vi "main_NI.vi"() -> ()   [LabVIEW 2017]
doc: "Эта версия для работы с системой сбора данных Agilent 34980A"
uses:
  <instrlib>/niDMM/nidmm.llb/niDMM Powerline Frequency.ctl
  <instrlib>/niDMM/nidmm.llb/niDMM Resolution in Digits.ctl
  <instrlib>/niDMM/nidmm.llb/niDMM Function.ctl
  <instrlib>/niDMM/nidmm.llb/niDMM Auto Zero.ctl
  <instrlib>/niDMM/nidmm.llb/niDMM ADC Calibration.ctl
  <vilib>/SwitchExecutive/nise.llb/niSE SessionRefnum.ctl
  <instrlib>/niDMM/nidmm.llb/niDMM Configure Measurement Digits.vi
  <vilib>/Utility/file.llb/Write Delimited Spreadsheet (string).vi
  VI/????????? ? ????????? ???????????? 34980A.vi
panel:
  in  "AllPlot":bool=TRUE caption="Все граф."
  out "Volt_3":dbl caption="V_3"
  in  "amountChip":i32=1 caption="Кол-во м/х" min=1 max=16 step=1
  out "isDMM":bool
  in  "DMM":refnum<k15>="-----"
  in  "wait befor meas, ms":u32=100 caption="Задержка ПЕРЕД\nизмерением, мс"
  out "ArrayTime 2":dbl[](array[numeric])
  out "Volt_2":dbl caption="V_2"
  out "Volt_1":dbl caption="V_1"
  in  "Emulate":bool
  out "ArrayOut":string[][](array[string])
  out "timer, s":dbl caption="Таймер, с"
  out "Waveform Graph":dbl[][](graph)
  in  "WaitAfterMeas, sec":u32 caption="Задержка ПОСЛЕ\nизм. всех приборов, с"
  in  "Record Data":bool
  out "error out":errorcluster
  in  "Save Button":bool
  # "В"
  # "В"
  # "В"
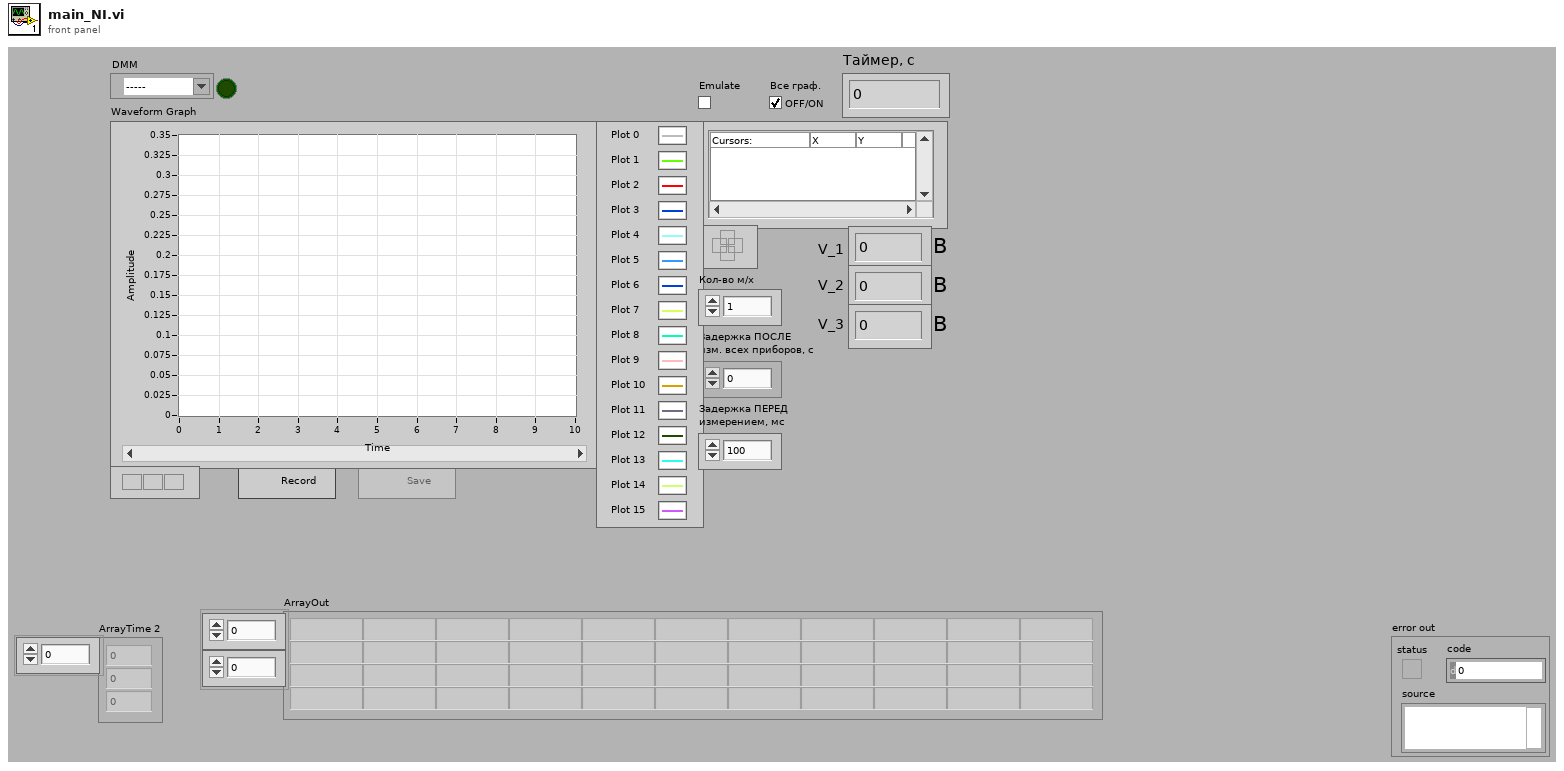
[diagram p1: front panel]
types:
  T1 = cluster{"Microchip_1":dbl[], "Microchip_2":dbl[], "Microchip_3":dbl[], "Microchip_4":dbl[], "Microchip_5":dbl[], "Microchip_6":dbl[], "Microchip_7":dbl[], "Microchip_8":dbl[], "Microchip_9":dbl[], "Microchip_10":dbl[], "Microchip_11":dbl[], "Microchip_12":dbl[], "Microchip_13":dbl[], "Microchip_14":dbl[], "Microchip_15":dbl[], "Microchip_16":dbl[]}
  T2 = enum8{"Enabled", "Disabled", "Disabled and Grayed Out"}
  T3 = typedef "niDMM Function.ctl" = enum16{"DC Volts", "AC Volts", "DC Current", "AC Current", "2-wire Resistance", "4-wire Resistance", "Diode", "Frequency", "Period", "AC Volts DC Coupled", "Capacitance", "Inductance", "Temperature"}
  T4 = typedef "niDMM Powerline Frequency.ctl" = enum16{"60 Hz", "50 Hz"}
  T5 = typedef "niDMM ADC Calibration.ctl" = i32
  T6 = typedef "niDMM Auto Zero.ctl" = i32
  T7 = typedef "niDMM Resolution in Digits.ctl" = dbl
  T8 = typedef "niSE SessionRefnum.ctl" = refnum<k1>
  T9 = cluster{"Microchip_1":string[], "Microchip_2":string[], "Microchip_3":string[], "Microchip_4":string[], "Microchip_5":string[], "Microchip_6":string[], "Microchip_7":string[], "Microchip_8":string[], "Microchip_9":string[], "Microchip_10":string[], "Microchip_11":string[], "Microchip_12":string[], "Microchip_13":string[], "Microchip_14":string[], "Microchip_15":string[], "Microchip_16":string[]}
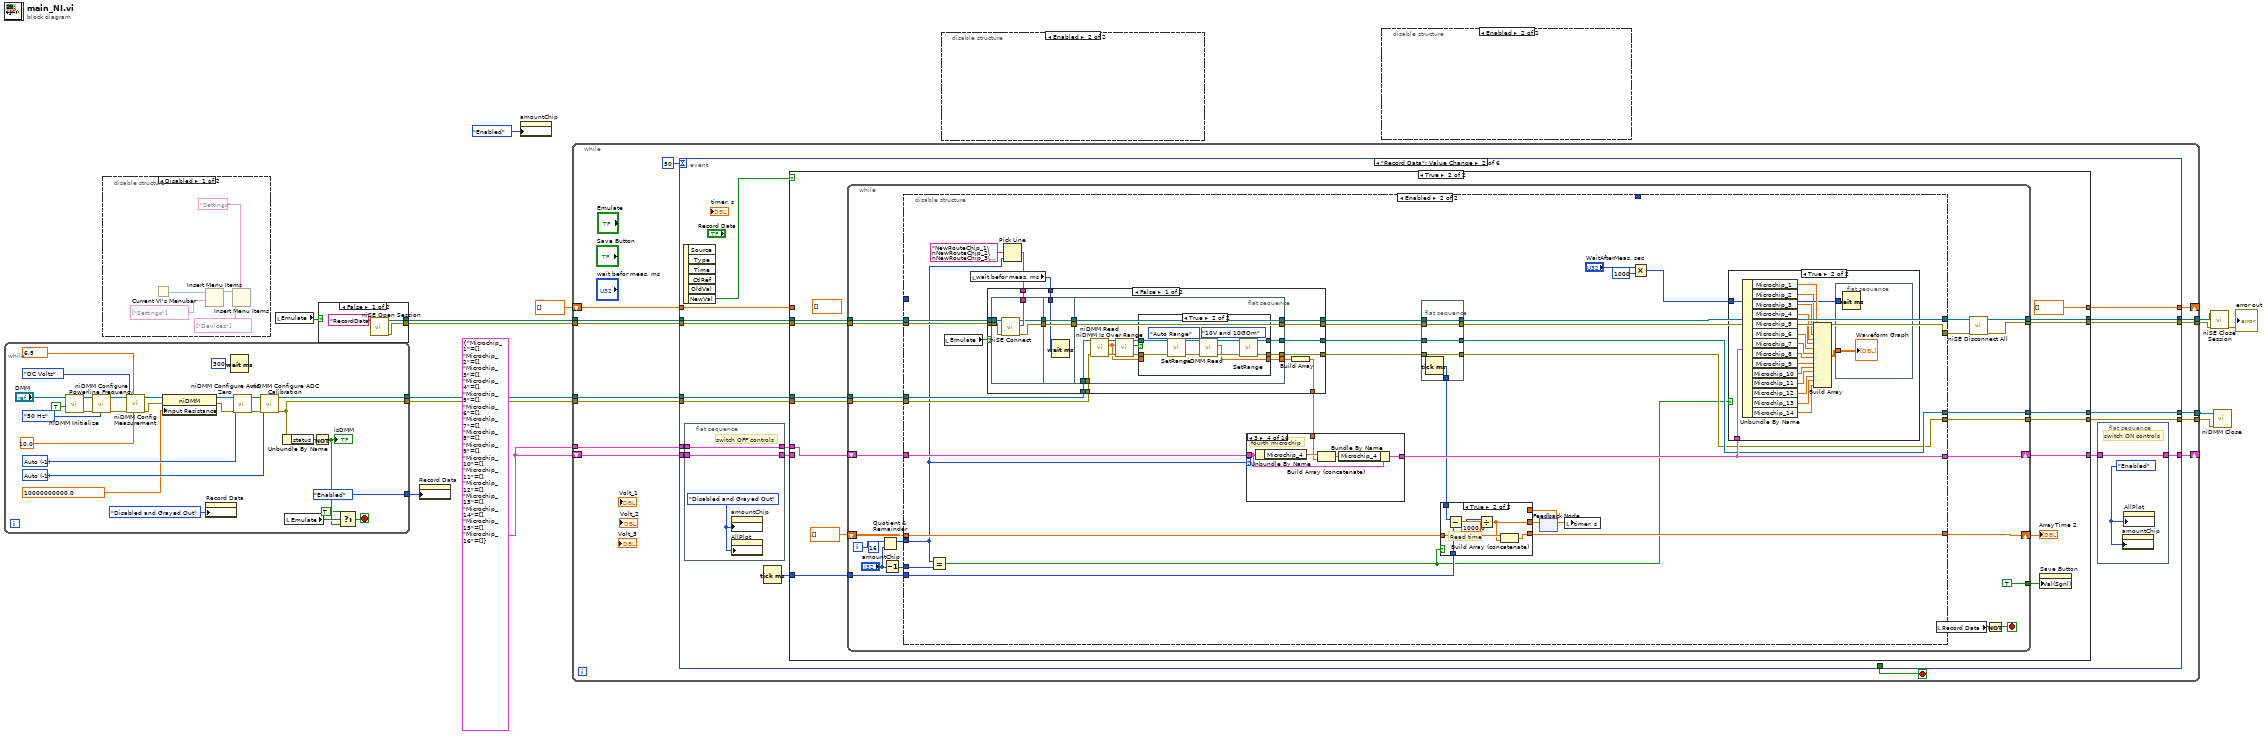
[diagram p0: block diagram]
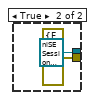
[diagram p2: hidden frame]
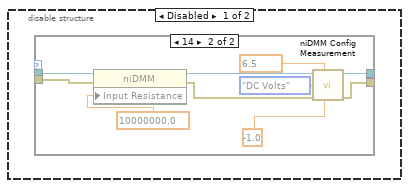
[diagram p3: hidden frame]
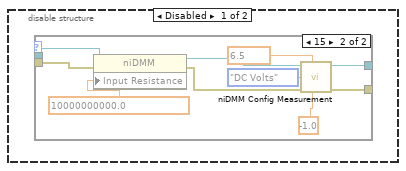
[diagram p5: hidden frame]
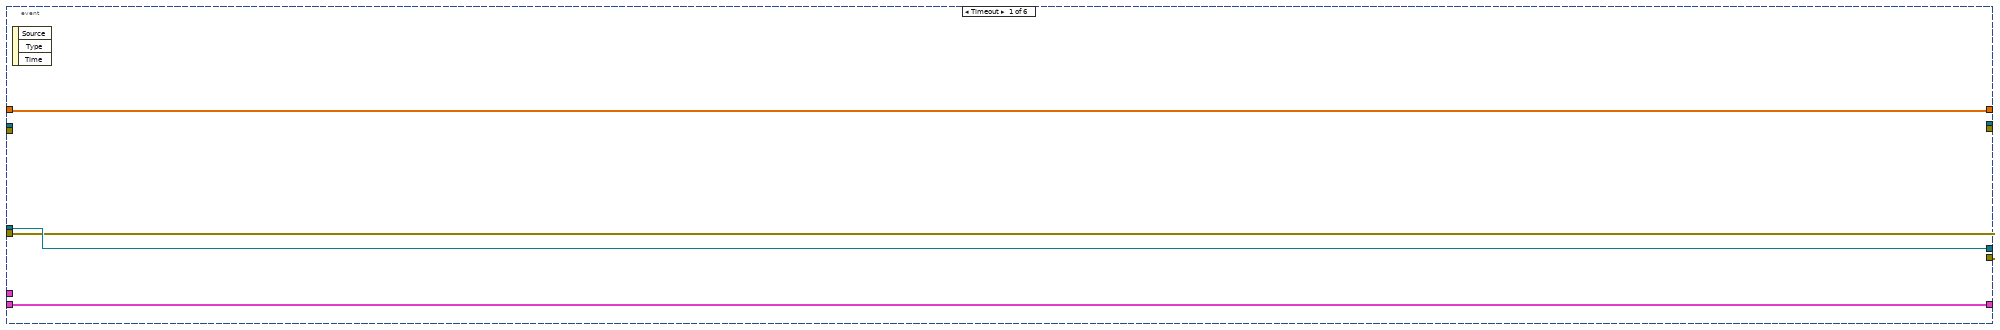
[diagram p8: hidden frame]
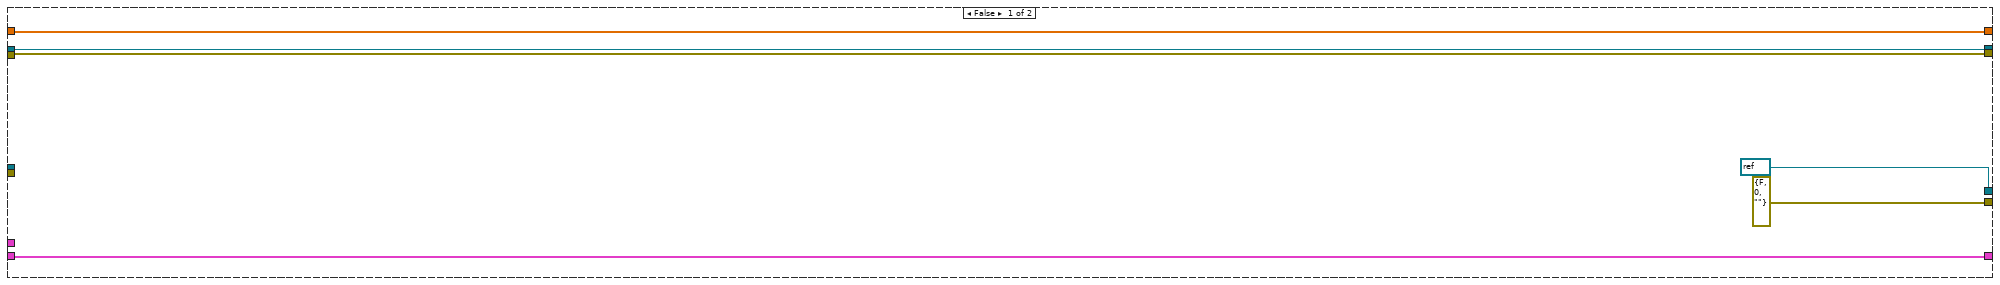
[diagram p9: hidden frame]
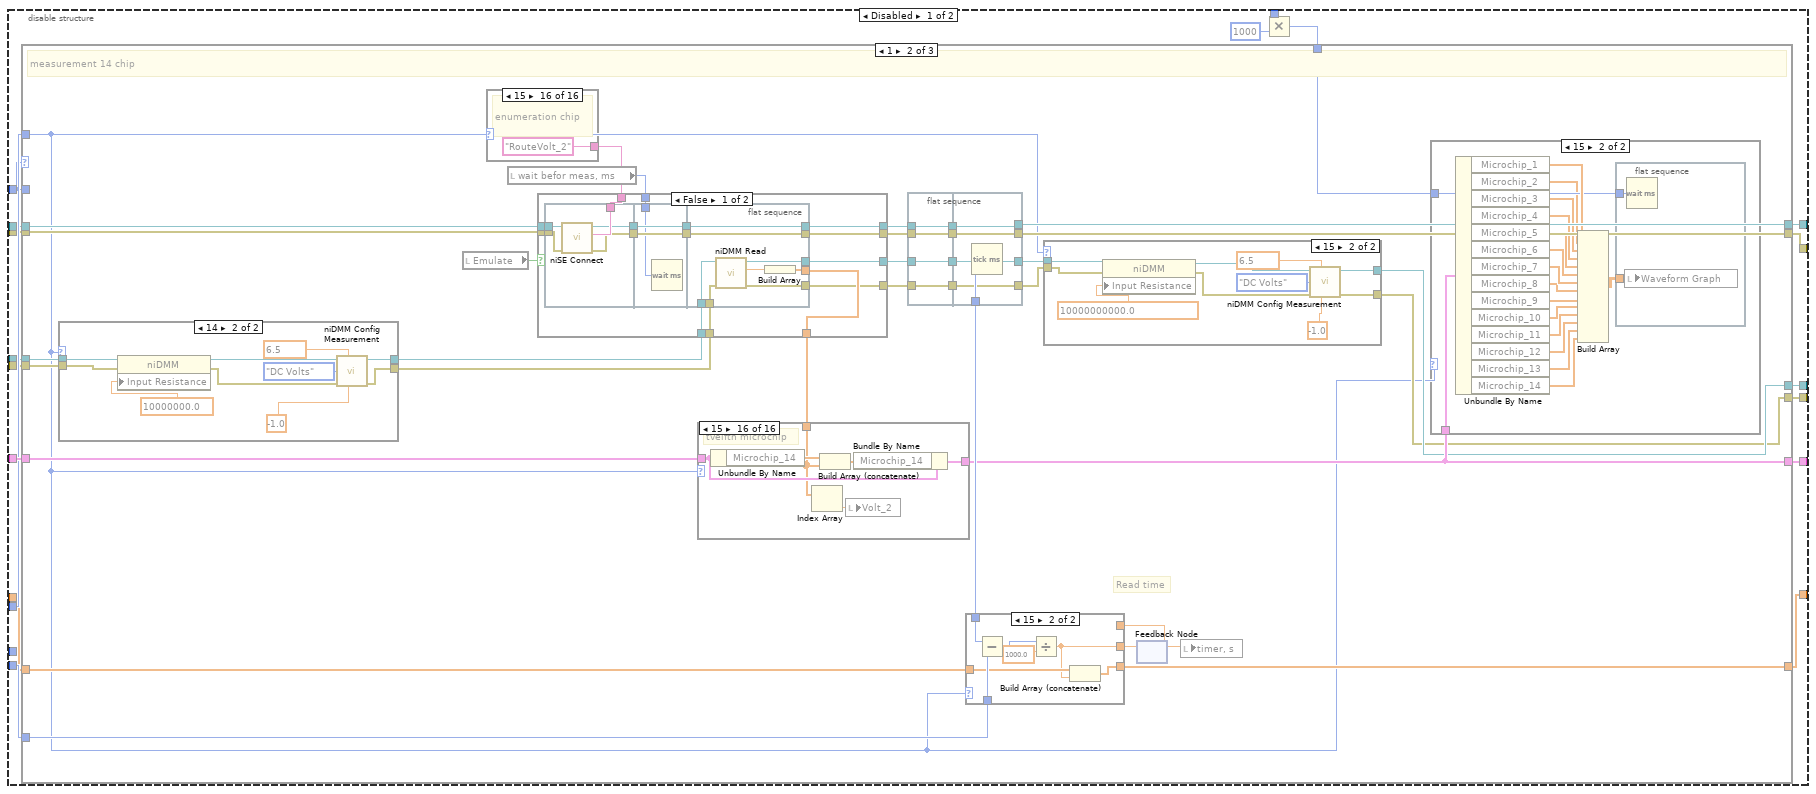
[diagram p10: hidden frame]
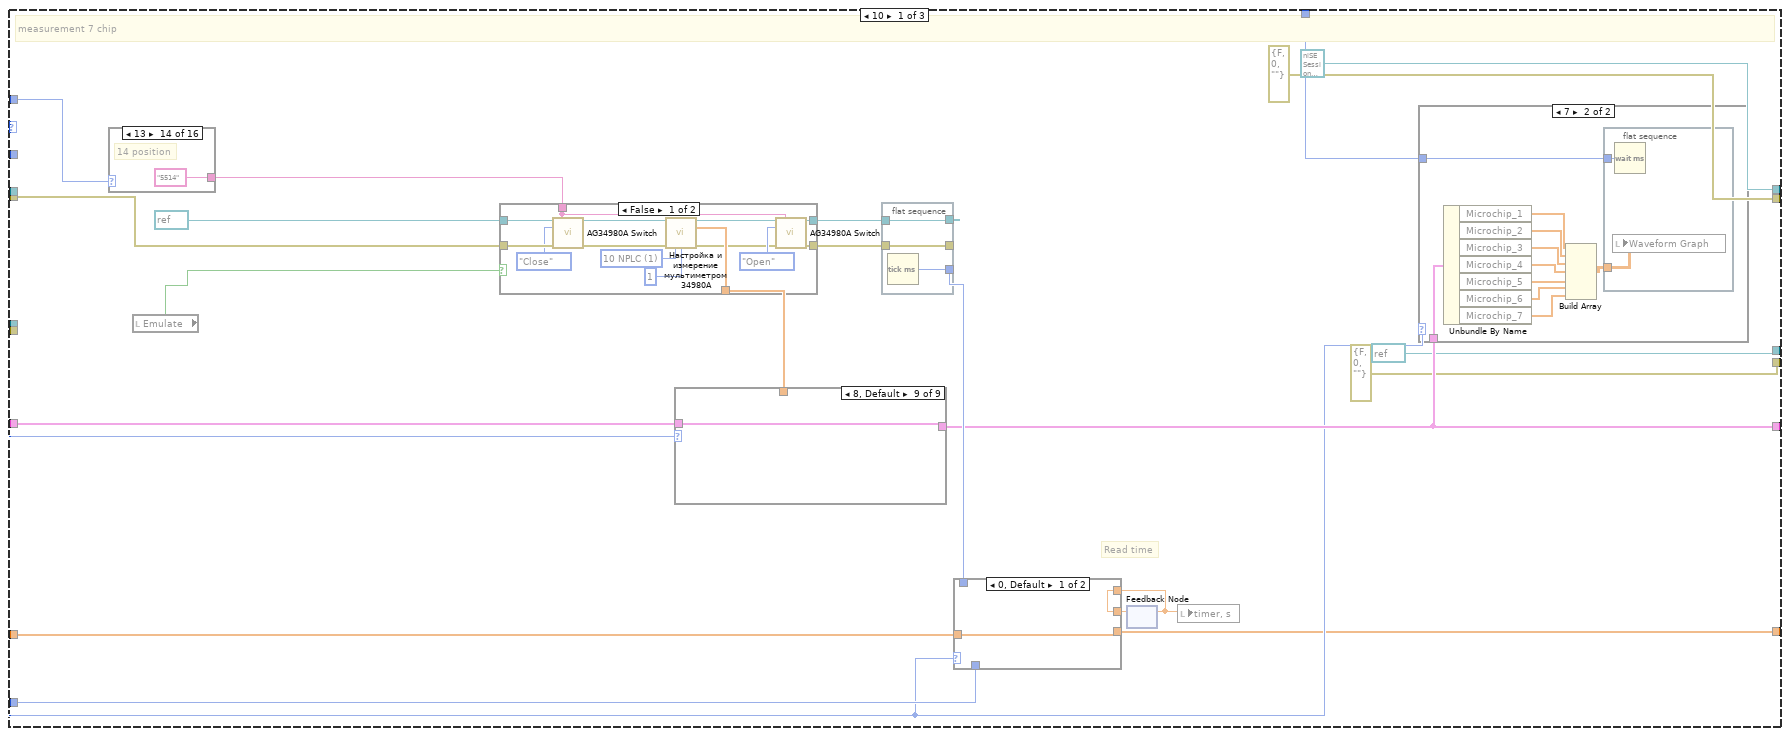
[diagram p11: hidden frame]
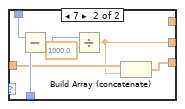
[diagram p13: hidden frame]
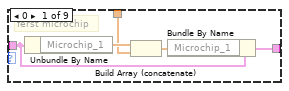
[diagram p14: hidden frame]
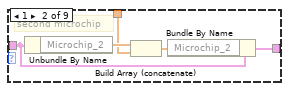
[diagram p15: hidden frame]
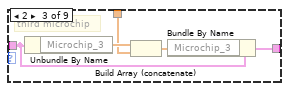
[diagram p16: hidden frame]
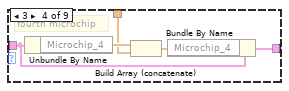
[diagram p17: hidden frame]
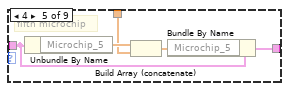
[diagram p18: hidden frame]
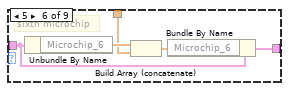
[diagram p19: hidden frame]
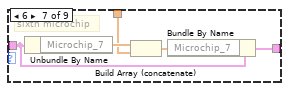
[diagram p20: hidden frame]
diagram:
  w13 = T1 {"Microchip_1"=[], "Microchip_2"=[], "Microchip_3"=[], "Microchip_4"=[], "Microchip_5"=[], "Microchip_6"=[], "Microchip_7"=[], "Microchip_8"=[], "Microchip_9"=[], "Microchip_10"=[], "Microchip_11"=[], "Microchip_12"=[], "Microchip_13"=[], "Microchip_14"=[], "Microchip_15"=[], "Microchip_16"=[]} ("Cluster Microchip")
  n1 = while {
    tunnel: [w34] -> w10
    tunnel: [w22] -> w9
    tunnel: [T2."Enabled" ("Disabled")] -> w3
    stop <- w16 stop-if-true
    w32 = 10000000000.0 items=["1 M Ohm"=1000000.0, "10 M Ohm"=10000000.0, "Greater Than 10 G Ohm"=10000000000.0] ("Configuration:Measurement Options:Input Resistance")
    w35 = T5 -1 items=["Auto"=-1, "Off"=0, "On"=1] ("ADC Calibration")
    w38 = T6 -1 items=["Auto"=-1, "Off"=0, "On"=1, "Once"=2] ("Auto Zero")
    w27 = T7 6.5 items=["3 1/2"=3.5, "4 1/2"=4.5, "5 1/2"=5.5, "6 1/2"=6.5, "7 1/2"=7.5] ("Resolution in Digits")
    n2 = call <instrlib>:"niDMM Initialize.vi"("Reset"=TRUE, "Instrument Descriptor"="DMM") -> ("error out"=w42:errorcluster, "instrument handle out"=w41:refnum<k15>)  [unwired: 8 in]
    n3 = call <instrlib>:"niDMM Configure Powerline Frequency.vi"("Powerline Frequency"=niDMM_Powerline_Frequency."50 Hz", "error in (no error)"=w42, "instrument handle"=w41) -> ("error out"=w25:errorcluster, "instrument handle out"=w26:refnum<k15>)  [unwired: 7 in]
    n4 = call-poly <instrlib>:"niDMM Config Measurement.vi"("Range"=10.0, "Resolution in Digits"=w27, "error in (no error)"=w25, "Function"=niDMM_Function."DC Volts", "instrument handle"=w26) -> ("error out"=w28:errorcluster, "instrument handle out"=w29:refnum<k15>)  [unwired: 5 in]
    n5 = property class="niDMM"(reference=w29, error in=w28, "Input Resistance"=w32) -> (reference out=w31:refnum<k15>, error out=w30:errorcluster)
    n6 = property on="Record Data" class="Bool (strict)"("DisabledEnum"=T2."Disabled and Grayed Out" ("Disabled")) -> ()  [unwired: 2 in, 2 out]
    n7 = Wait (ms)(milliseconds to wait=u32 300) -> ()  [unwired: 1 out]
    n8 = call <instrlib>:"niDMM Configure Auto Zero.vi"("error in (no error)"=w30, "Auto Zero"=w38, "instrument handle"=w31) -> ("error out"=w37:errorcluster, "instrument handle out"=w36:refnum<k15>)  [unwired: 7 in]
    n9 = call <instrlib>:"niDMM Configure ADC Calibration.vi"("error in (no error)"=w37, "ADC Calibration"=w35, "instrument handle"=w36) -> ("error out"=w22:errorcluster, "instrument handle out"=w34:refnum<k15>)  [unwired: 7 in]
    n10 = Unbundle By Name(w22) -> ("status"=w21:bool)
    n11 = local read "Emulate"() -> (w18:bool)
    n12 = Not(x=w21) -> (.not. x?=w17:bool)
    "isDMM" <- w17
    n13 = Select(t=TRUE, s=w18, f=w17) -> (s? t:f=w16:bool)
  }
  n14 = disable-structure shown="Disabled" {
    frame Disabled {
      n15 = Current VI's Menubar() -> (w47:refnum<k9>)
      n16 = Insert Menu Items(7:string[] ["Settings"] ("item tags"), 9:w47) -> (3:w46:refnum<k9>)  [unwired: 4 in, 2 out]
      n17 = Insert Menu Items(5:"Settings" ("menu tag"), 7:string[] ["Devices"] ("item tags"), 9:w46) -> ()  [unwired: 3 in, 3 out]
    }
    frame Enabled {
    }
  }
  n18 = local read "Emulate"() -> (w1:bool)
  n19 = case shown="False" w1 {
    tunnel: [w50 T8 refnum ("NISE Session (out)")] -> w12
    tunnel: [w49 errorcluster {"status"=FALSE, "code"=0, "source"=""} ("error out")] -> w11
    frame False {
      n20 = call <vilib>:"niSE Open Session.vi"("Virtual Device Name (SwitchConfiguration1)"="RecordData") -> ("error out"=w49:errorcluster, "NISE Session (out)"=w50:T8)  [unwired: 5 in]
    }
    frame True {
    }
  }
  n21 = property on="Record Data" class="Bool (strict)"("DisabledEnum"=w3) -> ()  [unwired: 2 in, 2 out]
  n22 = property on="amountChip" class="DigNum (strict)"("DisabledEnum"=T2."Enabled" ("Disabled")) -> ()  [unwired: 2 in, 2 out]
  n23 = while {
    shift-right: [w65] -> _
    shift-left: dbl[] [] -> [w66]
    shift-right: [w64] -> _
    shift-left: w13 -> [w63]
    tunnel: w13 -> [w62]
    tunnel: w12 -> [w61]
    tunnel: w11 -> [w60]
    tunnel: w10 -> [w59]
    tunnel: w9 -> [w56]
    tunnel: [w58] -> w8
    tunnel: [w57] -> w7
    tunnel: [w55] -> w5
    tunnel: [w54] -> w4
    stop <- w67 stop-if-true
    n24 = event shown="[1] \"Record Data\": Value Change" {
      selector: _ -> [_ _ _ _ _ _]
      dyn-events: _ -> [_ _ _ _ _ _]
      timeout: 50 -> [_ _ _ _ _ _]
      tunnel: [_ _ _ _ _ TRUE] -> w67
      tunnel: w66 -> [w71 w88 _ _ _ _]
      tunnel: [w71 w90 _ _ _ _] -> w65
      tunnel: w63 -> [w72 w85 w859 _ w893 w894]
      tunnel: [w72 w86 w859 _ w893 w894] -> w64
      tunnel: w62 -> [_ w83 _ _ _ _]
      tunnel: w61 -> [_ w80 _ _ _ _]
      tunnel: w60 -> [_ w79 _ _ _ _]
      tunnel: [_ w78 _ _ _ _] -> w57
      tunnel: [_ w77 _ _ _ _] -> w58
      tunnel: w59 -> [w70 w76 _ _ _ _]
      tunnel: w56 -> [w69 w75 _ _ _ _]
      tunnel: [w70 w74 _ _ _ _] -> w55
      tunnel: [w69 w73 _ _ _ _] -> w54
      event Timeout {
        n25 = event-data() -> ()  [unwired: 1 in, 3 out]
      }
      event "Record Data": Value Change {
        n26 = event-data() -> ("NewVal"=w81:bool)  [unwired: 1 in, 5 out]
        n27 = flat-sequence {
          tunnel: w85 -> [w93]
          tunnel: [w93] -> w84
          tunnel: w83 -> [w92]
          tunnel: [w92] -> w82
          frame #0 {
            w91 = T2."Disabled and Grayed Out" ("Disabled")
            # "switch OFF controls"
            n28 = property on="amountChip" class="DigNum (strict)"("DisabledEnum"=w91) -> ()  [unwired: 2 in, 2 out]
            n29 = property on="AllPlot" class="Bool (strict)"("DisabledEnum"=w91) -> ()  [unwired: 2 in, 2 out]
          }
        }
        n30 = Tick Count (ms)() -> (millisecond timer value=w89:u32)
        n31 = case shown="True" w81 {
          tunnel: w88 -> [w101 _]
          tunnel: [w101 dbl[] []] -> w90
          tunnel: w84 -> [w100 _]
          tunnel: [w100 w115] -> w87
          tunnel: w89 -> [_ w114]
          tunnel: w82 -> [_ w113]
          tunnel: w80 -> [w99 w112]
          tunnel: w79 -> [w98 w111]
          tunnel: [w99 w108] -> w78
          tunnel: [w98 w107] -> w77
          tunnel: w76 -> [_ w110]
          tunnel: w75 -> [_ w109]
          tunnel: [refnum<k15> refnum ("instrument handle out") w106] -> w74
          tunnel: [errorcluster {"status"=FALSE, "code"=0, "source"=""} ("error out") w105] -> w73
          frame False {
          }
          frame True {
            (unwired) dbl[] []
            n32 = while {
              shift-right: [w133] -> w115
              shift-left: w113 -> [w135]
              tunnel: w114 -> [w134]
              shift-right: [w130] -> w103
              shift-left: dbl[] [] ("ArrayTime 2") -> [w131]
              tunnel: w112 -> [w126]
              tunnel: w111 -> [w127]
              tunnel: w110 -> [w129]
              tunnel: w109 -> [w128]
              tunnel: [w123] -> w107
              tunnel: [w122] -> w108
              tunnel: [w121] -> w106
              tunnel: [w120] -> w105
              tunnel: [TRUE] -> w102
              i -> [w136]
              stop <- w137 stop-if-true
              (unwired) u32 16 ("y")
              n33 = Quotient & Remainder(x=w136, y="amountChip") -> (x-y*floor(x/y)=w132:i32)  [unwired: 1 out]
              n34 = Decrement(x="amountChip") -> (x-1=w118:i32)
              n35 = disable-structure shown="Enabled" {
                disable-tunnel: w135 -> [w156 w685]
                disable-tunnel: w134 -> [w155 w684]
                disable-tunnel: [w154 w683] -> w133
                disable-tunnel: w132 -> [w153 w671]
                disable-tunnel: w131 -> [w152 w682]
                disable-tunnel: [w151 w681] -> w130
                disable-tunnel: _ -> [w150 _]
                disable-tunnel: w129 -> [w149 w680]
                disable-tunnel: w128 -> [w148 w679]
                disable-tunnel: w127 -> [w147 w678]
                disable-tunnel: w126 -> [w146 w677]
                disable-tunnel: [w145 w676] -> w125
                disable-tunnel: [w144 w655] -> w124
                disable-tunnel: _ -> [w143 _]
                disable-tunnel: [w140 w673] -> w121
                disable-tunnel: [w139 w672] -> w120
                disable-tunnel: w118 -> [_ w670]
                frame Disabled {
                  n36 = Multiply(x=w143, y=u32 1000) -> (x*y=w141:u32)
                  n37 = case shown="1" w150 {
                    tunnel: w156 -> [w177 w311 w537]
                    tunnel: w155 -> [w172 w309 w536]
                    tunnel: [w170 w308 w535] -> w154
                    tunnel: w150 -> [_ _ _]
                    tunnel: w153 -> [w169 w279 w530]
                    tunnel: w152 -> [w168 w307 w534]
                    tunnel: [w167 w306 w533] -> w151
                    tunnel: w141 -> [w166 w305 w532]
                    tunnel: w149 -> [_ w287 w517]
                    tunnel: w148 -> [_ w286 w516]
                    tunnel: w147 -> [w161 w302 w513]
                    tunnel: w146 -> [_ w300 w514]
                    tunnel: [errorcluster {"status"=FALSE, "code"=0, "source"=""} ("error out") w291 w523] -> w145
                    tunnel: [T8 refnum ("NISE Session (out)") w298 w522] -> w144
                    tunnel: [refnum<k15> refnum ("instrument handle out") w281 w510] -> w140
                    tunnel: [errorcluster {"status"=FALSE, "code"=0, "source"=""} ("error out") w280 w509] -> w139
                    frame 10 {
                      # "Read time"
                      # "measurement 7 chip"
                      n38 = case shown="13" w169 {
                        tunnel: ["5501" ("Channel List") "5502" ("Channel List") "5503" ("Channel List") "5504" ("Channel List") "5505" ("Channel List") "5506" ("Channel List") "5507" ("Channel List") "5508" ("Channel List") "5509" ("Channel List") "5510" ("Channel List") "5511" ("Channel List") "5512" ("Channel List") "5513" ("Channel List") "5514" ("Channel List") "5515" ("Channel List") "5516" ("Channel List")] -> w175
                        frame 0, Default {
                          # "ferst position"
                        }
                        frame 1 {
                          # "second position"
                        }
                        frame 2 {
                          # "third position"
                        }
                        frame 3 {
                          # "fourth position"
                        }
                        frame 4 {
                          # "fifth position"
                        }
                        frame 5 {
                          # "sixth position"
                        }
                        frame 6 {
                          # "seventh position"
                        }
                        frame 7 {
                          # "eighth position"
                        }
                        frame 8 {
                          # "ninth position"
                        }
                        frame 9 {
                          # "tenth position"
                        }
                        frame 10 {
                          # "eleventh position"
                        }
                        frame 11 {
                          # "tvelfth position"
                        }
                        frame 12 {
                          # "13 position"
                        }
                        frame 13 {
                          # "14 position"
                        }
                        frame 14 {
                          # "15 position"
                        }
                        frame 15 {
                          # "16 position"
                        }
                      }
                      n39 = local read "Emulate"() -> (w165:bool)
                      n40 = case shown="False" w165 {
                        tunnel: refnum<visa-resource-name> refnum ("Commutator34980A") -> [w270 w271]
                        tunnel: [w269 w273] -> w176
                        tunnel: w175 -> [w268 _]
                        tunnel: [w267 w272] -> w174
                        tunnel: [w266 w271] -> w171
                        tunnel: w161 -> [w265 w272]
                        frame False {
                          w259 = u16 1 items=["1NPLC", "10 NPLC"] ("Скорост измерения")
                          n41 = call <instrlib>:"AG34980A Switch.vi"("VISA resource name"=w270, "Channel List"=w268, "Open/Close (0:Close)"=enum16{"Close", "Open"}."Close", "error in (no error)"=w265) -> ("VISA resource name out"=w258:refnum<visa-resource-name>, "error out"=w257:errorcluster)  [unwired: 9 in, 1 out]
                          n42 = call "Настройка и измерение мультиметром 34980A.vi"("Коммутатор Agilent 34980A in"=w258, "error in"=w257, "Скорост измерения"=w259, "Число измерений"=1) -> ("Коммутатор Agilent 34980A out"=w263:refnum<visa-resource-name>, "+U /-U выходное"=w269:dbl[], "error out 2"=w262:errorcluster)  [unwired: 9 in]
                          n43 = call <instrlib>:"AG34980A Switch.vi"("VISA resource name"=w263, "Channel List"=w268, "Open/Close (0:Close)"=enum16{"Close", "Open"}."Open", "error in (no error)"=w262) -> ("VISA resource name out"=w266:refnum<visa-resource-name>, "error out"=w267:errorcluster)  [unwired: 9 in, 1 out]
                        }
                        frame True {
                          n44 = Random Number (0-1)() -> (number: 0 to 1=w274:dbl)
                          n45 = Build Array(w274) -> (w273:dbl[])
                        }
                      }
                      n46 = case shown="8, Default" w169 {
                        tunnel: [w199 w204 w209 w214 w219 w224 w229 w236 w240] -> w170
                        tunnel: w177 -> [w200 w205 w210 w215 w220 w225 w230 w237 w240]
                        tunnel: w176 -> [w202 w207 w212 w217 w222 w227 w232 w235 _]
                        frame 0 {
                          # "ferst microchip"
                          n47 = Unbundle By Name(w200) -> ("Microchip_1"=w203:dbl[])
                          n48 = Build Array (concatenate)(w203, w202) -> (w201:dbl[])
                          n49 = Bundle By Name(cluster=w200, "Microchip_1"=w201) -> (w199:T1)
                        }
                        frame 1 {
                          # "second microchip"
                          n50 = Unbundle By Name(w205) -> ("Microchip_2"=w208:dbl[])
                          n51 = Build Array (concatenate)(w208, w207) -> (w206:dbl[])
                          n52 = Bundle By Name(cluster=w205, "Microchip_2"=w206) -> (w204:T1)
                        }
                        frame 2 {
                          # "third microchip"
                          n53 = Unbundle By Name(w210) -> ("Microchip_3"=w213:dbl[])
                          n54 = Build Array (concatenate)(w213, w212) -> (w211:dbl[])
                          n55 = Bundle By Name(cluster=w210, "Microchip_3"=w211) -> (w209:T1)
                        }
                        frame 3 {
                          # "fourth microchip"
                          n56 = Unbundle By Name(w215) -> ("Microchip_4"=w218:dbl[])
                          n57 = Build Array (concatenate)(w218, w217) -> (w216:dbl[])
                          n58 = Bundle By Name(cluster=w215, "Microchip_4"=w216) -> (w214:T1)
                        }
                        frame 4 {
                          # "fifth microchip"
                          n59 = Unbundle By Name(w220) -> ("Microchip_5"=w223:dbl[])
                          n60 = Build Array (concatenate)(w223, w222) -> (w221:dbl[])
                          n61 = Bundle By Name(cluster=w220, "Microchip_5"=w221) -> (w219:T1)
                        }
                        frame 5 {
                          # "sixth microchip"
                          n62 = Unbundle By Name(w225) -> ("Microchip_6"=w228:dbl[])
                          n63 = Build Array (concatenate)(w228, w227) -> (w226:dbl[])
                          n64 = Bundle By Name(cluster=w225, "Microchip_6"=w226) -> (w224:T1)
                        }
                        frame 6 {
                          # "sixth microchip"
                          n65 = Unbundle By Name(w230) -> ("Microchip_7"=w233:dbl[])
                          n66 = Build Array (concatenate)(w233, w232) -> (w231:dbl[])
                          n67 = Bundle By Name(cluster=w230, "Microchip_7"=w231) -> (w229:T1)
                        }
                        frame 7 {
                          # "sixth microchip"
                          n68 = Unbundle By Name(w237) -> ("Microchip_14"=w239:dbl[])
                          n69 = Index Array(array=w235) -> (element=w234:dbl)  [unwired: 1 in]
                          n70 = Build Array (concatenate)(w239, w235) -> (w238:dbl[])
                          n71 = local write "Volt_1"(w234) -> ()
                          n72 = Bundle By Name(cluster=w237, "Microchip_14"=w238) -> (w236:T1)
                        }
                        frame 8, Default {
                        }
                      }
                      n73 = flat-sequence {
                        tunnel: w174 -> [w277]
                        tunnel: [w277] -> _
                        tunnel: [w276] -> w173
                        tunnel: w171 -> [w275]
                        tunnel: [w275] -> _
                        frame #0 {
                          n74 = Tick Count (ms)() -> (millisecond timer value=w276:u32)
                        }
                      }
                      n75 = feedback #1() -> (w160:dbl)  [unwired: 1 in]
                      n76 = case shown="0, Default" w169 {
                        tunnel: w173 -> [_ w198]
                        tunnel: w172 -> [_ w197]
                        tunnel: [w191 w195] -> w167
                        tunnel: w168 -> [w191 w196]
                        tunnel: [w190 w192] -> w164
                        tunnel: w160 -> [w190 _]
                        frame 0, Default {
                        }
                        frame 7 {
                          n77 = Subtract(x=w198, y=w197) -> (x-y=w194:u32)
                          n78 = Divide(x=w194, y=1000.0) -> (x/y=w192:dbl)
                          n79 = Build Array (concatenate)(w196, w192) -> (w195:dbl[])
                        }
                      }
                      n80 = feedback-in #1(w164) -> ()
                      n81 = local write "timer, s"(w160) -> ()
                      n82 = case shown="7" w169 {
                        tunnel: w170 -> [_ w184]
                        tunnel: w166 -> [_ w185]
                        frame 0, Default {
                        }
                        frame 7 {
                          n83 = Unbundle By Name(w184) -> ("Microchip_1"=w187:dbl[], "Microchip_2"=w183:dbl[], "Microchip_3"=w182:dbl[], "Microchip_4"=w181:dbl[], "Microchip_5"=w180:dbl[], "Microchip_6"=w179:dbl[], "Microchip_7"=w178:dbl[])
                          n84 = Build Array(w187, w183, w182, w181, w180, w179, w178) -> (w186:dbl[][])
                          n85 = flat-sequence {
                            tunnel: w186 -> [w189]
                            tunnel: w185 -> [w188]
                            frame #0 {
                              n86 = local write "Waveform Graph"(w189) -> ()
                              n87 = Wait (ms)(milliseconds to wait=w188) -> ()  [unwired: 1 out]
                            }
                          }
                        }
                      }
                    }
                    frame 1 {
                      # "Read time"
                      # "measurement 14 chip"
                      n88 = case shown="14" w279 {
                        tunnel: w287 -> [w325 w334]
                        tunnel: w286 -> [w324 w333]
                        tunnel: [w325 w327] -> w285
                        tunnel: [w324 w326] -> w284
                        frame 0, Default {
                        }
                        frame 14 {
                          w331 = T7 6.5 items=["3 1/2"=3.5, "4 1/2"=4.5, "5 1/2"=5.5, "6 1/2"=6.5, "7 1/2"=7.5] ("Resolution in Digits")
                          w335 = 10000000.0 items=["1 M Ohm"=1000000.0, "10 M Ohm"=10000000.0, "Greater Than 10 G Ohm"=10000000000.0] ("Configuration:Measurement Options:Input Resistance")
                          n89 = property class="niDMM"(reference=w334, error in=w333, "Input Resistance"=w335) -> (reference out=w329:refnum<k15>, error out=w328:errorcluster)
                          n90 = call-poly <instrlib>:"niDMM Config Measurement.vi"("Range"=-1.0, "Resolution in Digits"=w331, "error in (no error)"=w328, "Function"=niDMM_Function."DC Volts", "instrument handle"=w329) -> ("error out"=w326:errorcluster, "instrument handle out"=w327:refnum<k15>)  [unwired: 5 in]
                        }
                      }
                      n91 = local read "Emulate"() -> (w304:bool)
                      n92 = case shown="15" w279 {
                        tunnel: ["RouteChip_1" ("Connection Specification (\"\")") "RouteChip_2" ("Connection Specification (\"\")") "RouteChip_3" ("Connection Specification (\"\")") "RouteChip_4" ("Connection Specification (\"\")") "RouteChip_5" ("Connection Specification (\"\")") "RouteChip_6" ("Connection Specification (\"\")") "RouteChip_7" ("Connection Specification (\"\")") "RouteChip_8" ("Connection Specification (\"\")") "RouteChip_9" ("Connection Specification (\"\")") "RouteChip_10" ("Connection Specification (\"\")") "RouteChip_11" ("Connection Specification (\"\")") "RouteChip_12" ("Connection Specification (\"\")") "RouteChip_13" ("Connection Specification (\"\")") "RouteChip_14" ("Connection Specification (\"\")") "RouteVolt_1" ("Connection Specification (\"\")") "RouteVolt_2" ("Connection Specification (\"\")")] -> w301
                        frame 0, Default {
                          # "enumeration chip"
                        }
                        frame 1 {
                          # "enumeration chip"
                        }
                        frame 2 {
                          # "enumeration chip"
                        }
                        frame 3 {
                          # "enumeration chip"
                        }
                        frame 4 {
                          # "enumeration chip"
                        }
                        frame 5 {
                          # "enumeration chip"
                        }
                        frame 6 {
                          # "enumeration chip"
                        }
                        frame 7 {
                          # "enumeration chip"
                        }
                        frame 8 {
                          # "enumeration chip"
                        }
                        frame 9 {
                          # "enumeration chip"
                        }
                        frame 10 {
                          # "enumeration chip"
                        }
                        frame 11 {
                          # "enumeration chip"
                        }
                        frame 12 {
                          # "enumeration chip"
                        }
                        frame 13 {
                          # "enumeration chip"
                        }
                        frame 14 {
                          # "enumeration chip"
                        }
                        frame 15 {
                          # "enumeration chip"
                        }
                      }
                      n93 = local read "wait befor meas, ms"() -> (w278:u32)
                      n94 = case shown="False" w304 {
                        tunnel: w302 -> [w476 w495]
                        tunnel: w301 -> [w475 _]
                        tunnel: w300 -> [w474 w497]
                        tunnel: [w473 w497] -> w299
                        tunnel: [w464 w494] -> w289
                        tunnel: w285 -> [w465 w496]
                        tunnel: w284 -> [w466 w494]
                        tunnel: [w463 w496] -> w288
                        tunnel: [w472 w495] -> w292
                        tunnel: [w467 w493] -> w290
                        tunnel: w278 -> [w462 _]
                        frame False {
                          n95 = flat-sequence {
                            tunnel: w476 -> [w481]
                            tunnel: w475 -> [w480]
                            tunnel: w474 -> [w479]
                            tunnel: [w478] -> w471
                            tunnel: [w477] -> w470
                            tunnel: w471 -> [w484]
                            tunnel: w470 -> [w483]
                            tunnel: [w484] -> w469
                            tunnel: [w483] -> w468
                            tunnel: w462 -> [w482]
                            tunnel: [w491] -> w472
                            tunnel: [w492] -> w473
                            tunnel: w469 -> [w492]
                            tunnel: w468 -> [w491]
                            tunnel: [w489] -> w467
                            tunnel: [w488] -> w464
                            tunnel: [w487] -> w463
                            tunnel: w466 -> [w486]
                            tunnel: w465 -> [w485]
                            frame #0 {
                              n96 = call <vilib>:"niSE Connect.vi"("error in (no error)"=w481, "Connection Specification (\"\")"=w480, "NISE Session (in)"=w479) -> ("error out"=w477:errorcluster, "NISE Session (out)"=w478:T8)  [unwired: 7 in]
                            }
                            frame #1 {
                              n97 = Wait (ms)(milliseconds to wait=w482) -> ()  [unwired: 1 out]
                            }
                            frame #2 {
                              n98 = call <instrlib>:"niDMM Read.vi"("error in (no error)"=w486, "instrument handle"=w485) -> ("error out"=w488:errorcluster, "Measurement"=w490:dbl, "instrument handle out"=w487:refnum<k15>)  [unwired: 7 in]
                              n99 = Build Array(w490) -> (w489:dbl[])
                            }
                          }
                        }
                        frame True {
                          n100 = Random Number (0-1)() -> (number: 0 to 1=w498:dbl)
                          n101 = Build Array(w498) -> (w493:dbl[])
                        }
                      }
                      n102 = case shown="15" w279 {
                        tunnel: [w380 w385 w390 w395 w400 w405 w410 w415 w420 w425 w430 w435 w440 w445 w452 w458] -> w308
                        tunnel: w311 -> [w381 w386 w391 w396 w401 w406 w411 w416 w421 w426 w431 w436 w441 w446 w453 w459]
                        tunnel: w290 -> [w383 w388 w393 w398 w403 w408 w413 w418 w423 w428 w433 w438 w443 w448 w451 w457]
                        frame 0, Default {
                          # "ferst microchip"
                          n103 = Unbundle By Name(w381) -> ("Microchip_1"=w384:dbl[])
                          n104 = Build Array (concatenate)(w384, w383) -> (w382:dbl[])
                          n105 = Bundle By Name(cluster=w381, "Microchip_1"=w382) -> (w380:T1)
                        }
                        frame 1 {
                          # "second microchip"
                          n106 = Unbundle By Name(w386) -> ("Microchip_2"=w389:dbl[])
                          n107 = Build Array (concatenate)(w389, w388) -> (w387:dbl[])
                          n108 = Bundle By Name(cluster=w386, "Microchip_2"=w387) -> (w385:T1)
                        }
                        frame 2 {
                          # "third microchip"
                          n109 = Unbundle By Name(w391) -> ("Microchip_3"=w394:dbl[])
                          n110 = Build Array (concatenate)(w394, w393) -> (w392:dbl[])
                          n111 = Bundle By Name(cluster=w391, "Microchip_3"=w392) -> (w390:T1)
                        }
                        frame 3 {
                          # "fourth microchip"
                          n112 = Unbundle By Name(w396) -> ("Microchip_4"=w399:dbl[])
                          n113 = Build Array (concatenate)(w399, w398) -> (w397:dbl[])
                          n114 = Bundle By Name(cluster=w396, "Microchip_4"=w397) -> (w395:T1)
                        }
                        frame 4 {
                          # "fifth microchip"
                          n115 = Unbundle By Name(w401) -> ("Microchip_5"=w404:dbl[])
                          n116 = Build Array (concatenate)(w404, w403) -> (w402:dbl[])
                          n117 = Bundle By Name(cluster=w401, "Microchip_5"=w402) -> (w400:T1)
                        }
                        frame 5 {
                          # "sixth microchip"
                          n118 = Unbundle By Name(w406) -> ("Microchip_6"=w409:dbl[])
                          n119 = Build Array (concatenate)(w409, w408) -> (w407:dbl[])
                          n120 = Bundle By Name(cluster=w406, "Microchip_6"=w407) -> (w405:T1)
                        }
                        frame 6 {
                          # "seventh microchip"
                          n121 = Unbundle By Name(w411) -> ("Microchip_7"=w414:dbl[])
                          n122 = Build Array (concatenate)(w414, w413) -> (w412:dbl[])
                          n123 = Bundle By Name(cluster=w411, "Microchip_7"=w412) -> (w410:T1)
                        }
                        frame 7 {
                          # "eighth microchip"
                          n124 = Unbundle By Name(w416) -> ("Microchip_8"=w419:dbl[])
                          n125 = Build Array (concatenate)(w419, w418) -> (w417:dbl[])
                          n126 = Bundle By Name(cluster=w416, "Microchip_8"=w417) -> (w415:T1)
                        }
                        frame 8 {
                          # "ninth microchip"
                          n127 = Unbundle By Name(w421) -> ("Microchip_9"=w424:dbl[])
                          n128 = Build Array (concatenate)(w424, w423) -> (w422:dbl[])
                          n129 = Bundle By Name(cluster=w421, "Microchip_9"=w422) -> (w420:T1)
                        }
                        frame 9 {
                          # "tenth microchip"
                          n130 = Unbundle By Name(w426) -> ("Microchip_10"=w429:dbl[])
                          n131 = Build Array (concatenate)(w429, w428) -> (w427:dbl[])
                          n132 = Bundle By Name(cluster=w426, "Microchip_10"=w427) -> (w425:T1)
                        }
                        frame 10 {
                          # "eleventh microchip"
                          n133 = Unbundle By Name(w431) -> ("Microchip_11"=w434:dbl[])
                          n134 = Build Array (concatenate)(w434, w433) -> (w432:dbl[])
                          n135 = Bundle By Name(cluster=w431, "Microchip_11"=w432) -> (w430:T1)
                        }
                        frame 11 {
                          # "tvelfth microchip"
                          n136 = Unbundle By Name(w436) -> ("Microchip_12"=w439:dbl[])
                          n137 = Build Array (concatenate)(w439, w438) -> (w437:dbl[])
                          n138 = Bundle By Name(cluster=w436, "Microchip_12"=w437) -> (w435:T1)
                        }
                        frame 12 {
                          # "tvelfth microchip"
                          n139 = Unbundle By Name(w441) -> ("Microchip_13"=w444:dbl[])
                          n140 = Build Array (concatenate)(w444, w443) -> (w442:dbl[])
                          n141 = Bundle By Name(cluster=w441, "Microchip_13"=w442) -> (w440:T1)
                        }
                        frame 13 {
                          # "tvelfth microchip"
                          n142 = Unbundle By Name(w446) -> ("Microchip_14"=w449:dbl[])
                          n143 = Build Array (concatenate)(w449, w448) -> (w447:dbl[])
                          n144 = Bundle By Name(cluster=w446, "Microchip_14"=w447) -> (w445:T1)
                        }
                        frame 14 {
                          # "tvelfth microchip"
                          n145 = Unbundle By Name(w453) -> ("Microchip_14"=w455:dbl[])
                          n146 = Index Array(array=w451) -> (element=w450:dbl)  [unwired: 1 in]
                          n147 = Build Array (concatenate)(w455, w451) -> (w454:dbl[])
                          n148 = local write "Volt_1"(w450) -> ()
                          n149 = Bundle By Name(cluster=w453, "Microchip_14"=w454) -> (w452:T1)
                        }
                        frame 15 {
                          # "tvelfth microchip"
                          n150 = Unbundle By Name(w459) -> ("Microchip_14"=w461:dbl[])
                          n151 = Index Array(array=w457) -> (element=w456:dbl)  [unwired: 1 in]
                          n152 = Build Array (concatenate)(w461, w457) -> (w460:dbl[])
                          n153 = local write "Volt_2"(w456) -> ()
                          n154 = Bundle By Name(cluster=w459, "Microchip_14"=w460) -> (w458:T1)
                        }
                      }
                      n155 = flat-sequence {
                        tunnel: w289 -> [w501]
                        tunnel: w299 -> [w502]
                        tunnel: [w502] -> w297
                        tunnel: [w501] -> w296
                        tunnel: [w500] -> w294
                        tunnel: w288 -> [w500]
                        tunnel: [w499] -> w293
                        tunnel: w292 -> [w499]
                        tunnel: [w507] -> w310
                        tunnel: [w506] -> w298
                        tunnel: [w505] -> w282
                        tunnel: w297 -> [w506]
                        tunnel: w296 -> [w505]
                        tunnel: w294 -> [w504]
                        tunnel: [w504] -> w283
                        tunnel: w293 -> [w503]
                        tunnel: [w503] -> w291
                        frame #0 {
                        }
                        frame #1 {
                          n156 = Tick Count (ms)() -> (millisecond timer value=w507:u32)
                        }
                      }
                      n157 = case shown="15" w279 {
                        tunnel: w283 -> [w313 w322]
                        tunnel: w282 -> [w312 w321]
                        tunnel: [w313 w315] -> w281
                        tunnel: [w312 w314] -> w280
                        frame 0, Default {
                        }
                        frame 15 {
                          w319 = T7 6.5 items=["3 1/2"=3.5, "4 1/2"=4.5, "5 1/2"=5.5, "6 1/2"=6.5, "7 1/2"=7.5] ("Resolution in Digits")
                          w323 = 10000000000.0 items=["1 M Ohm"=1000000.0, "10 M Ohm"=10000000.0, "Greater Than 10 G Ohm"=10000000000.0] ("Configuration:Measurement Options:Input Resistance")
                          n158 = property class="niDMM"(reference=w322, error in=w321, "Input Resistance"=w323) -> (reference out=w317:refnum<k15>, error out=w316:errorcluster)
                          n159 = call-poly <instrlib>:"niDMM Config Measurement.vi"("Range"=-1.0, "Resolution in Digits"=w319, "error in (no error)"=w316, "Function"=niDMM_Function."DC Volts", "instrument handle"=w317) -> ("error out"=w314:errorcluster, "instrument handle out"=w315:refnum<k15>)  [unwired: 5 in]
                        }
                      }
                      n160 = feedback #2() -> (w295:dbl)  [unwired: 1 in]
                      n161 = case shown="15" w279 {
                        tunnel: w310 -> [_ w379]
                        tunnel: w309 -> [_ w378]
                        tunnel: [w372 w376] -> w306
                        tunnel: w307 -> [w372 w377]
                        tunnel: [w371 w373] -> w303
                        tunnel: w295 -> [w371 _]
                        frame 0, Default {
                        }
                        frame 15 {
                          n162 = Subtract(x=w379, y=w378) -> (x-y=w375:u32)
                          n163 = Divide(x=w375, y=1000.0) -> (x/y=w373:dbl)
                          n164 = Build Array (concatenate)(w377, w373) -> (w376:dbl[])
                        }
                      }
                      n165 = feedback-in #2(w303) -> ()
                      n166 = local write "timer, s"(w295) -> ()
                      n167 = case shown="15" w279 {
                        tunnel: w308 -> [_ w366]
                        tunnel: w305 -> [_ w365]
                        frame 0, Default {
                        }
                        frame 15 {
                          n168 = Unbundle By Name(w366) -> ("Microchip_1"=w368:dbl[], "Microchip_2"=w364:dbl[], "Microchip_3"=w363:dbl[], "Microchip_4"=w362:dbl[], "Microchip_5"=w361:dbl[], "Microchip_6"=w360:dbl[], "Microchip_7"=w359:dbl[], "Microchip_8"=w358:dbl[], "Microchip_9"=w357:dbl[], "Microchip_10"=w356:dbl[], "Microchip_11"=w355:dbl[], "Microchip_12"=w354:dbl[], "Microchip_13"=w353:dbl[], "Microchip_14"=w352:dbl[])
                          n169 = Build Array(w368, w364, w363, w362, w361, w360, w359, w358, w357, w356, w355, w354, w353, w352) -> (w367:dbl[][])
                          n170 = flat-sequence {
                            tunnel: w367 -> [w370]
                            tunnel: w365 -> [w369]
                            frame #0 {
                              n171 = local write "Waveform Graph"(w370) -> ()
                              n172 = Wait (ms)(milliseconds to wait=w369) -> ()  [unwired: 1 out]
                            }
                          }
                        }
                      }
                    }
                    frame 0, Default {
                      # "Read time"
                      # "measurement 7 chip"
                      n173 = local read "Emulate"() -> (w515:bool)
                      n174 = case shown="7" w530 {
                        tunnel: ["RouteChip_1" ("Connection Specification (\"\")") "RouteChip_2" ("Connection Specification (\"\")") "RouteChip_3" ("Connection Specification (\"\")") "RouteChip_4" ("Connection Specification (\"\")") "RouteChip_5" ("Connection Specification (\"\")") "RouteChip_6" ("Connection Specification (\"\")") "RouteChip_7" ("Connection Specification (\"\")") "RouteVolt_1" ("Connection Specification (\"\")")] -> w512
                        frame 0, Default {
                          # "enumeration chip"
                        }
                        frame 1 {
                          # "enumeration chip"
                        }
                        frame 2 {
                          # "enumeration chip"
                        }
                        frame 3 {
                          # "enumeration chip"
                        }
                        frame 4 {
                          # "enumeration chip"
                        }
                        frame 5 {
                          # "enumeration chip"
                        }
                        frame 6 {
                          # "enumeration chip"
                        }
                        frame 7 {
                          # "enumeration chip"
                        }
                      }
                      n175 = local read "wait befor meas, ms"() -> (w508:u32)
                      n176 = case shown="False" w515 {
                        tunnel: w513 -> [w552 w571]
                        tunnel: w512 -> [w551 _]
                        tunnel: w514 -> [w550 w573]
                        tunnel: [w549 w573] -> w519
                        tunnel: [w540 w570] -> w520
                        tunnel: w517 -> [w541 w572]
                        tunnel: w516 -> [w542 w570]
                        tunnel: [w539 w572] -> w521
                        tunnel: [w548 w571] -> w518
                        tunnel: [w543 w569] -> w511
                        tunnel: w508 -> [w538 _]
                        frame False {
                          n177 = flat-sequence {
                            tunnel: w552 -> [w557]
                            tunnel: w551 -> [w556]
                            tunnel: w550 -> [w555]
                            tunnel: [w554] -> w547
                            tunnel: [w553] -> w546
                            tunnel: w547 -> [w560]
                            tunnel: w546 -> [w559]
                            tunnel: [w560] -> w545
                            tunnel: [w559] -> w544
                            tunnel: w538 -> [w558]
                            tunnel: [w567] -> w548
                            tunnel: [w568] -> w549
                            tunnel: w545 -> [w568]
                            tunnel: w544 -> [w567]
                            tunnel: [w565] -> w543
                            tunnel: [w564] -> w540
                            tunnel: [w563] -> w539
                            tunnel: w542 -> [w562]
                            tunnel: w541 -> [w561]
                            frame #0 {
                              n178 = call <vilib>:"niSE Connect.vi"("error in (no error)"=w557, "Connection Specification (\"\")"=w556, "NISE Session (in)"=w555) -> ("error out"=w553:errorcluster, "NISE Session (out)"=w554:T8)  [unwired: 7 in]
                            }
                            frame #1 {
                              n179 = Wait (ms)(milliseconds to wait=w558) -> ()  [unwired: 1 out]
                            }
                            frame #2 {
                              n180 = call <instrlib>:"niDMM Read.vi"("error in (no error)"=w562, "instrument handle"=w561) -> ("error out"=w564:errorcluster, "Measurement"=w566:dbl, "instrument handle out"=w563:refnum<k15>)  [unwired: 7 in]
                              n181 = Build Array(w566) -> (w565:dbl[])
                            }
                          }
                        }
                        frame True {
                          n182 = Random Number (0-1)() -> (number: 0 to 1=w574:dbl)
                          n183 = Build Array(w574) -> (w569:dbl[])
                        }
                      }
                      n184 = case shown="7" w530 {
                        tunnel: [w613 w618 w623 w628 w633 w638 w643 w650 w654] -> w535
                        tunnel: w537 -> [w614 w619 w624 w629 w634 w639 w644 w651 w654]
                        tunnel: w511 -> [w616 w621 w626 w631 w636 w641 w646 w649 _]
                        frame 0 {
                          # "ferst microchip"
                          n185 = Unbundle By Name(w614) -> ("Microchip_1"=w617:dbl[])
                          n186 = Build Array (concatenate)(w617, w616) -> (w615:dbl[])
                          n187 = Bundle By Name(cluster=w614, "Microchip_1"=w615) -> (w613:T1)
                        }
                        frame 1 {
                          # "second microchip"
                          n188 = Unbundle By Name(w619) -> ("Microchip_2"=w622:dbl[])
                          n189 = Build Array (concatenate)(w622, w621) -> (w620:dbl[])
                          n190 = Bundle By Name(cluster=w619, "Microchip_2"=w620) -> (w618:T1)
                        }
                        frame 2 {
                          # "third microchip"
                          n191 = Unbundle By Name(w624) -> ("Microchip_3"=w627:dbl[])
                          n192 = Build Array (concatenate)(w627, w626) -> (w625:dbl[])
                          n193 = Bundle By Name(cluster=w624, "Microchip_3"=w625) -> (w623:T1)
                        }
                        frame 3 {
                          # "fourth microchip"
                          n194 = Unbundle By Name(w629) -> ("Microchip_4"=w632:dbl[])
                          n195 = Build Array (concatenate)(w632, w631) -> (w630:dbl[])
                          n196 = Bundle By Name(cluster=w629, "Microchip_4"=w630) -> (w628:T1)
                        }
                        frame 4 {
                          # "fifth microchip"
                          n197 = Unbundle By Name(w634) -> ("Microchip_5"=w637:dbl[])
                          n198 = Build Array (concatenate)(w637, w636) -> (w635:dbl[])
                          n199 = Bundle By Name(cluster=w634, "Microchip_5"=w635) -> (w633:T1)
                        }
                        frame 5 {
                          # "sixth microchip"
                          n200 = Unbundle By Name(w639) -> ("Microchip_6"=w642:dbl[])
                          n201 = Build Array (concatenate)(w642, w641) -> (w640:dbl[])
                          n202 = Bundle By Name(cluster=w639, "Microchip_6"=w640) -> (w638:T1)
                        }
                        frame 6 {
                          # "seventh microchip"
                          n203 = Unbundle By Name(w644) -> ("Microchip_7"=w647:dbl[])
                          n204 = Build Array (concatenate)(w647, w646) -> (w645:dbl[])
                          n205 = Bundle By Name(cluster=w644, "Microchip_7"=w645) -> (w643:T1)
                        }
                        frame 7 {
                          # "tvelfth microchip"
                          n206 = Unbundle By Name(w651) -> ("Microchip_14"=w653:dbl[])
                          n207 = Index Array(array=w649) -> (element=w648:dbl)  [unwired: 1 in]
                          n208 = Build Array (concatenate)(w653, w649) -> (w652:dbl[])
                          n209 = local write "Volt_1"(w648) -> ()
                          n210 = Bundle By Name(cluster=w651, "Microchip_14"=w652) -> (w650:T1)
                        }
                        frame 8, Default {
                        }
                      }
                      n211 = flat-sequence {
                        tunnel: w520 -> [w577]
                        tunnel: w519 -> [w578]
                        tunnel: [w578] -> w528
                        tunnel: [w577] -> w527
                        tunnel: [w576] -> w526
                        tunnel: w521 -> [w576]
                        tunnel: [w575] -> w525
                        tunnel: w518 -> [w575]
                        tunnel: [w583] -> w524
                        tunnel: [w582] -> w509
                        tunnel: w528 -> [w579]
                        tunnel: w527 -> [w582]
                        tunnel: w526 -> [w581]
                        tunnel: [w581] -> w510
                        tunnel: w525 -> [w580]
                        tunnel: [w580] -> w523
                        tunnel: [w579] -> w522
                        frame #0 {
                        }
                        frame #1 {
                          n212 = Tick Count (ms)() -> (millisecond timer value=w583:u32)
                        }
                      }
                      n213 = feedback #3() -> (w529:dbl)  [unwired: 1 in]
                      n214 = case shown="7" w530 {
                        tunnel: w524 -> [_ w612]
                        tunnel: w536 -> [_ w611]
                        tunnel: [w605 w609] -> w533
                        tunnel: w534 -> [w605 w610]
                        tunnel: [w604 w606] -> w531
                        tunnel: w529 -> [w604 _]
                        frame 0, Default {
                        }
                        frame 7 {
                          n215 = Subtract(x=w612, y=w611) -> (x-y=w608:u32)
                          n216 = Divide(x=w608, y=1000.0) -> (x/y=w606:dbl)
                          n217 = Build Array (concatenate)(w610, w606) -> (w609:dbl[])
                        }
                      }
                      n218 = feedback-in #3(w531) -> ()
                      n219 = local write "timer, s"(w529) -> ()
                      n220 = case shown="15" w530 {
                        tunnel: w535 -> [_ w599]
                        tunnel: w532 -> [_ w598]
                        frame 0, Default {
                        }
                        frame 15 {
                          n221 = Unbundle By Name(w599) -> ("Microchip_1"=w601:dbl[], "Microchip_2"=w597:dbl[], "Microchip_3"=w596:dbl[], "Microchip_4"=w595:dbl[], "Microchip_5"=w594:dbl[], "Microchip_6"=w593:dbl[], "Microchip_7"=w592:dbl[])
                          n222 = Build Array(w601, w597, w596, w595, w594, w593, w592) -> (w600:dbl[][])
                          n223 = flat-sequence {
                            tunnel: w600 -> [w603]
                            tunnel: w598 -> [w602]
                            frame #0 {
                              n224 = local write "Waveform Graph"(w603) -> ()
                              n225 = Wait (ms)(milliseconds to wait=w602) -> ()  [unwired: 1 out]
                            }
                          }
                        }
                      }
                    }
                  }
                }
                frame Enabled {
                  # "Read time"
                  n226 = Equal?(x=w671, y=w670) -> (x = y?=w657:bool)
                  n227 = local read "Emulate"() -> (w667:bool)
                  n228 = local read "wait befor meas, ms"() -> (w659:u32)
                  n229 = Pick Line(multi-line string="NewRouteChip_1\nNewRouteChip_2\nNewRouteChip_3\nNewRouteChip_4\nNewRouteChip_5\nNewRouteChip_6\nNewRouteChip_7\nNewRouteChip_8\nNewRouteChip_9\nNewRouteChip_10\nNewRouteChip_11\nNewRouteChip_12\nNewRouteChip_13\nNewRouteChip_14\nNewRouteChip_15\nNewRouteChip_16", line index=w671) -> (output string=w658:string)  [unwired: 1 in]
                  n230 = case shown="False" w667 {
                    tunnel: w678 -> [w812 w850]
                    tunnel: w658 -> [w811 _]
                    tunnel: w677 -> [w810 w852]
                    tunnel: [w809 w852] -> w665
                    tunnel: [w801 w849] -> w661
                    tunnel: w680 -> [w802 w851]
                    tunnel: w679 -> [w803 w849]
                    tunnel: [w800 w851] -> w660
                    tunnel: [w808 w850] -> w663
                    tunnel: [w797 w848] -> w662
                    tunnel: w659 -> [w799 _]
                    frame False {
                      n231 = flat-sequence {
                        tunnel: w812 -> [w817]
                        tunnel: w811 -> [w816]
                        tunnel: w810 -> [w815]
                        tunnel: [w814] -> w807
                        tunnel: [w813] -> w806
                        tunnel: w807 -> [w820]
                        tunnel: w806 -> [w819]
                        tunnel: [w820] -> w805
                        tunnel: [w819] -> w804
                        tunnel: w799 -> [w818]
                        tunnel: [w832] -> w808
                        tunnel: [w833] -> w809
                        tunnel: w805 -> [w833]
                        tunnel: w804 -> [w832]
                        tunnel: [w824] -> w801
                        tunnel: [w823] -> w800
                        tunnel: w803 -> [w831]
                        tunnel: w802 -> [w830]
                        tunnel: [w822] -> w798
                        frame #0 {
                          n232 = call <vilib>:"niSE Connect.vi"("error in (no error)"=w817, "Connection Specification (\"\")"=w816, "NISE Session (in)"=w815) -> ("error out"=w813:errorcluster, "NISE Session (out)"=w814:T8)  [unwired: 7 in]
                        }
                        frame #1 {
                          n233 = Wait (ms)(milliseconds to wait=w818) -> ()  [unwired: 1 out]
                        }
                        frame #2 {
                          n234 = call <instrlib>:"niDMM Read.vi"("error in (no error)"=w831, "instrument handle"=w830) -> ("error out"=w828:errorcluster, "Measurement"=w821:dbl, "instrument handle out"=w829:refnum<k15>)  [unwired: 7 in]
                          n235 = call <instrlib>:"niDMM Is Over Range.vi"("error in (no error)"=w828, "Measurement"=w821, "instrument handle"=w829) -> ("error out"=w825:errorcluster, "Over Range?"=w827:bool, "instrument handle out"=w826:refnum<k15>)  [unwired: 6 in]
                          n236 = case shown="True" w827 {
                            tunnel: w826 -> [w836 w847]
                            tunnel: w825 -> [w835 w846]
                            tunnel: [w836 w839] -> w823
                            tunnel: [w835 w838] -> w824
                            tunnel: [w834 w837] -> w822
                            tunnel: w821 -> [w834 _]
                            frame False {
                            }
                            frame True {
                              n237 = call "SetRange.vi"("Enum"=enum16{"Auto Range", "10V and 10GOm"}."Auto Range", "error in"=w846, "instrument handle in"=w847) -> ("error out"=w843:errorcluster, "instrument handle out"=w844:refnum<k15>)  [unwired: 7 in]
                              n238 = call <instrlib>:"niDMM Read.vi"("error in (no error)"=w843, "instrument handle"=w844) -> ("error out"=w841:errorcluster, "Measurement"=w837:dbl, "instrument handle out"=w842:refnum<k15>)  [unwired: 7 in]
                              n239 = call "SetRange.vi"("Enum"=enum16{"Auto Range", "10V and 10GOm"}."10V and 10GOm", "error in"=w841, "instrument handle in"=w842) -> ("error out"=w838:errorcluster, "instrument handle out"=w839:refnum<k15>)  [unwired: 7 in]
                            }
                          }
                        }
                      }
                      n240 = Build Array(w798) -> (w797:dbl[])
                    }
                    frame True {
                      n241 = Random Number (0-1)() -> (number: 0 to 1=w853:dbl)
                      n242 = Build Array(w853) -> (w848:dbl[])
                    }
                  }
                  n243 = case shown="3" w671 {
                    tunnel: [w716 w722 w728 w732 w737 w742 w747 w752 w757 w762 w767 w772 w777 w782 w788 w793] -> w683
                    tunnel: w685 -> [w717 w723 w729 w733 w738 w743 w748 w753 w758 w763 w768 w773 w778 w783 w789 w794]
                    tunnel: w662 -> [w714 w720 w726 w735 w740 w745 w750 w755 w760 w765 w770 w775 w780 w785 w787 w792]
                    frame 0, Default {
                      # "ferst microchip"
                      n244 = Unbundle By Name(w717) -> ("Microchip_1"=w719:dbl[])
                      n245 = Index Array(array=w714) -> (element=w715:dbl)  [unwired: 1 in]
                      n246 = Build Array (concatenate)(w719, w714) -> (w718:dbl[])
                      n247 = local write "Volt_1"(w715) -> ()
                      n248 = Bundle By Name(cluster=w717, "Microchip_1"=w718) -> (w716:T1)
                    }
                    frame 1 {
                      # "second microchip"
                      n249 = Unbundle By Name(w723) -> ("Microchip_2"=w725:dbl[])
                      n250 = Index Array(array=w720) -> (element=w721:dbl)  [unwired: 1 in]
                      n251 = Build Array (concatenate)(w725, w720) -> (w724:dbl[])
                      n252 = local write "Volt_2"(w721) -> ()
                      n253 = Bundle By Name(cluster=w723, "Microchip_2"=w724) -> (w722:T1)
                    }
                    frame 2 {
                      # "third microchip"
                      n254 = Unbundle By Name(w729) -> ("Microchip_3"=w731:dbl[])
                      n255 = Index Array(array=w726) -> (element=w727:dbl)  [unwired: 1 in]
                      n256 = Build Array (concatenate)(w731, w726) -> (w730:dbl[])
                      n257 = local write "Volt_3"(w727) -> ()
                      n258 = Bundle By Name(cluster=w729, "Microchip_3"=w730) -> (w728:T1)
                    }
                    frame 3 {
                      # "fourth microchip"
                      n259 = Unbundle By Name(w733) -> ("Microchip_4"=w736:dbl[])
                      n260 = Build Array (concatenate)(w736, w735) -> (w734:dbl[])
                      n261 = Bundle By Name(cluster=w733, "Microchip_4"=w734) -> (w732:T1)
                    }
                    frame 4 {
                      # "fifth microchip"
                      n262 = Unbundle By Name(w738) -> ("Microchip_5"=w741:dbl[])
                      n263 = Build Array (concatenate)(w741, w740) -> (w739:dbl[])
                      n264 = Bundle By Name(cluster=w738, "Microchip_5"=w739) -> (w737:T1)
                    }
                    frame 5 {
                      # "sixth microchip"
                      n265 = Unbundle By Name(w743) -> ("Microchip_6"=w746:dbl[])
                      n266 = Build Array (concatenate)(w746, w745) -> (w744:dbl[])
                      n267 = Bundle By Name(cluster=w743, "Microchip_6"=w744) -> (w742:T1)
                    }
                    frame 6 {
                      # "seventh microchip"
                      n268 = Unbundle By Name(w748) -> ("Microchip_7"=w751:dbl[])
                      n269 = Build Array (concatenate)(w751, w750) -> (w749:dbl[])
                      n270 = Bundle By Name(cluster=w748, "Microchip_7"=w749) -> (w747:T1)
                    }
                    frame 7 {
                      # "eighth microchip"
                      n271 = Unbundle By Name(w753) -> ("Microchip_8"=w756:dbl[])
                      n272 = Build Array (concatenate)(w756, w755) -> (w754:dbl[])
                      n273 = Bundle By Name(cluster=w753, "Microchip_8"=w754) -> (w752:T1)
                    }
                    frame 8 {
                      # "ninth microchip"
                      n274 = Unbundle By Name(w758) -> ("Microchip_9"=w761:dbl[])
                      n275 = Build Array (concatenate)(w761, w760) -> (w759:dbl[])
                      n276 = Bundle By Name(cluster=w758, "Microchip_9"=w759) -> (w757:T1)
                    }
                    frame 9 {
                      # "tenth microchip"
                      n277 = Unbundle By Name(w763) -> ("Microchip_10"=w766:dbl[])
                      n278 = Build Array (concatenate)(w766, w765) -> (w764:dbl[])
                      n279 = Bundle By Name(cluster=w763, "Microchip_10"=w764) -> (w762:T1)
                    }
                    frame 10 {
                      # "eleventh microchip"
                      n280 = Unbundle By Name(w768) -> ("Microchip_11"=w771:dbl[])
                      n281 = Build Array (concatenate)(w771, w770) -> (w769:dbl[])
                      n282 = Bundle By Name(cluster=w768, "Microchip_11"=w769) -> (w767:T1)
                    }
                    frame 11 {
                      # "tvelfth microchip"
                      n283 = Unbundle By Name(w773) -> ("Microchip_12"=w776:dbl[])
                      n284 = Build Array (concatenate)(w776, w775) -> (w774:dbl[])
                      n285 = Bundle By Name(cluster=w773, "Microchip_12"=w774) -> (w772:T1)
                    }
                    frame 12 {
                      # "tvelfth microchip"
                      n286 = Unbundle By Name(w778) -> ("Microchip_13"=w781:dbl[])
                      n287 = Build Array (concatenate)(w781, w780) -> (w779:dbl[])
                      n288 = Bundle By Name(cluster=w778, "Microchip_13"=w779) -> (w777:T1)
                    }
                    frame 13 {
                      # "tvelfth microchip"
                      n289 = Unbundle By Name(w783) -> ("Microchip_14"=w786:dbl[])
                      n290 = Build Array (concatenate)(w786, w785) -> (w784:dbl[])
                      n291 = Bundle By Name(cluster=w783, "Microchip_14"=w784) -> (w782:T1)
                    }
                    frame 14 {
                      # "tvelfth microchip"
                      n292 = Unbundle By Name(w789) -> ("Microchip_15"=w791:dbl[])
                      n293 = Build Array (concatenate)(w791, w787) -> (w790:dbl[])
                      n294 = Bundle By Name(cluster=w789, "Microchip_15"=w790) -> (w788:T1)
                    }
                    frame 15 {
                      # "tvelfth microchip"
                      n295 = Unbundle By Name(w794) -> ("Microchip_16"=w796:dbl[])
                      n296 = Build Array (concatenate)(w796, w792) -> (w795:dbl[])
                      n297 = Bundle By Name(cluster=w794, "Microchip_16"=w795) -> (w793:T1)
                    }
                  }
                  n298 = flat-sequence {
                    tunnel: [w858] -> w668
                    tunnel: [w857] -> w655
                    tunnel: [w856] -> w672
                    tunnel: [w855] -> w673
                    tunnel: [w854] -> w676
                    tunnel: w665 -> [w857]
                    tunnel: w661 -> [w856]
                    tunnel: w660 -> [w855]
                    tunnel: w663 -> [w854]
                    frame #0 {
                      n299 = Tick Count (ms)() -> (millisecond timer value=w858:u32)
                    }
                  }
                  n300 = feedback #4() -> (w664:dbl)  [unwired: 1 in]
                  n301 = case shown="True" w657 {
                    tunnel: w668 -> [_ w713]
                    tunnel: w684 -> [_ w712]
                    tunnel: [w706 w710] -> w681
                    tunnel: w682 -> [w706 w711]
                    tunnel: [w705 w707] -> w666
                    tunnel: w664 -> [w705 _]
                    frame False {
                    }
                    frame True {
                      n302 = Subtract(x=w713, y=w712) -> (x-y=w709:u32)
                      n303 = Divide(x=w709, y=1000.0) -> (x/y=w707:dbl)
                      n304 = Build Array (concatenate)(w711, w707) -> (w710:dbl[])
                    }
                  }
                  n305 = feedback-in #4(w666) -> ()
                  n306 = local write "timer, s"(w664) -> ()
                  n307 = Multiply(x="WaitAfterMeas, sec", y=u32 1000) -> (x*y=w674:u32)
                  n308 = case shown="True" w657 {
                    tunnel: w683 -> [_ w700]
                    tunnel: w674 -> [_ w699]
                    frame False {
                    }
                    frame True {
                      n309 = Unbundle By Name(w700) -> ("Microchip_1"=w702:dbl[], "Microchip_2"=w698:dbl[], "Microchip_3"=w697:dbl[], "Microchip_4"=w696:dbl[], "Microchip_5"=w695:dbl[], "Microchip_6"=w694:dbl[], "Microchip_7"=w693:dbl[], "Microchip_8"=w692:dbl[], "Microchip_9"=w691:dbl[], "Microchip_10"=w690:dbl[], "Microchip_11"=w689:dbl[], "Microchip_12"=w688:dbl[], "Microchip_13"=w687:dbl[], "Microchip_14"=w686:dbl[])
                      n310 = Build Array(w702, w698, w697, w696, w695, w694, w693, w692, w691, w690, w689, w688, w687, w686) -> (w701:dbl[][])
                      n311 = flat-sequence {
                        tunnel: w701 -> [w703]
                        tunnel: w699 -> [w704]
                        frame #0 {
                          n312 = Wait (ms)(milliseconds to wait=w704) -> ()  [unwired: 1 out]
                          "Waveform Graph" <- w703
                        }
                      }
                    }
                  }
                }
              }
              n313 = local read "Record Data"() -> (w138:bool)
              n314 = call <vilib>:"niSE Disconnect All.vi"("error in (no error)"=w125, "NISE Session (in)"=w124) -> ("error out"=w123:errorcluster, "NISE Session (out)"=w122:T8)  [unwired: 4 in]
              n315 = Not(x=w138) -> (.not. x?=w137:bool)
            }
            "ArrayTime 2" <- w103
            n316 = property on="Save Button" class="Bool (strict)"("Val(Sgnl)"=w102) -> ()  [unwired: 2 in, 2 out]
          }
        }
        n317 = flat-sequence {
          tunnel: w87 -> [w95]
          tunnel: [w95] -> w86
          frame #0 {
            w94 = T2."Enabled" ("Disabled")
            # "switch ON controls"
            n318 = property on="amountChip" class="DigNum (strict)"("DisabledEnum"=w94) -> ()  [unwired: 2 in, 2 out]
            n319 = property on="AllPlot" class="Bool (strict)"("DisabledEnum"=w94) -> ()  [unwired: 2 in, 2 out]
          }
        }
      }
      event "Save Button": Value Change {
        n320 = event-data() -> ()  [unwired: 1 in, 6 out]
        n321 = flat-sequence {
          tunnel: w859 -> [w883]
          frame #0 {
            n322 = call "ReadDecimal.vi"() -> ("Флаг Разделителя"=w885:bool)  [unwired: 11 in]
            n323 = call "PathToRezult.vi"() -> ("pathToRezult"=w884:path)  [unwired: 11 in]
            n324 = Number To Fractional String(use system decimal point (T)=w885, number=w883) -> (F-format string=w882:T9)  [unwired: 2 in]
            n325 = Unbundle By Name(w882) -> ("Microchip_1"=w875:string[], "Microchip_2"=w874:string[], "Microchip_3"=w873:string[], "Microchip_4"=w872:string[], "Microchip_5"=w871:string[], "Microchip_6"=w870:string[], "Microchip_7"=w869:string[], "Microchip_8"=w868:string[], "Microchip_9"=w867:string[], "Microchip_10"=w866:string[], "Microchip_11"=w865:string[], "Microchip_12"=w864:string[], "Microchip_13"=w863:string[], "Microchip_14"=w862:string[], "Microchip_15"=w861:string[], "Microchip_16"=w860:string[])
            n326 = local read "ArrayTime 2"() -> (w881:dbl[])
            n327 = Number To Fractional String(use system decimal point (T)=w885, number=w881) -> (F-format string=w880:string[])  [unwired: 2 in]
            n328 = Build Array(w875, w874, w873, w872, w871, w870, w869, w868, w867, w866, w865, w864, w863, w862, w861, w860) -> (w879:string[][])
            n329 = Build Array (concatenate)(w880) -> (w878:string[])
            n330 = Build Array (concatenate)(w878, w879) -> (w877:string[][])
            n331 = Transpose 2D Array(2D array=w877) -> (transposed array=w876:string[][])
            "ArrayOut" <- w876
            n332 = call-poly <vilib>:"Write Delimited Spreadsheet.vi"("file path (dialog if empty)"=w884, "2D data"=w876) -> ()  [unwired: 12 in, 2 out]
          }
          frame #1 {
            n333 = local write "Save Button"(FALSE ("Save Button")) -> ()
          }
        }
      }
      event "AllPlot": Value Change {
        n334 = event-data() -> ("NewVal"=w888:bool)  [unwired: 1 in, 5 out]
        n335 = for {
          N: 16 -> [_]
          tunnel: w888 -> [w890]
          i -> [w891]
          n336 = property on="Waveform Graph" class="WFGraph (strict)"("Active Plot"=w891) -> (error out=w889:errorcluster)  [unwired: 2 in, 1 out]
          n337 = property on="Waveform Graph" class="WFGraph (strict)"(error in=w889, "Plot.Visible?"=w890) -> ()  [unwired: 1 in, 2 out]
        }
      }
      event Menu Selection (User) {
        n338 = event-data() -> ("ItemTag"=w892:string)  [unwired: 1 in, 6 out]
        n339 = case shown="\"SwitchImage\"" w892 {
          frame "False", Default {
          }
          frame "SwitchImage" {
            n340 = call "HelpSwitchMatrix.vi"() -> ()  [unwired: 12 in]
          }
        }
      }
      event Application Instance Close; Panel Close {
        n341 = event-data() -> ()  [unwired: 1 in, 3 out]
        n342 = One Button Dialog(message="Кирдык") -> ()  [unwired: 1 in, 1 out]
      }
    }
  }
  n343 = disable-structure shown="Enabled" {
    frame Disabled {
      n344 = case shown="14" {
        selector: _ -> [_ _]
        tunnel: _ -> [w898 w907]
        tunnel: _ -> [w897 w906]
        tunnel: [w898 w900] -> _
        tunnel: [w897 w899] -> _
        frame 0, Default {
        }
        frame 14 {
          w904 = T7 6.5 items=["3 1/2"=3.5, "4 1/2"=4.5, "5 1/2"=5.5, "6 1/2"=6.5, "7 1/2"=7.5] ("Resolution in Digits")
          w908 = 10000000.0 items=["1 M Ohm"=1000000.0, "10 M Ohm"=10000000.0, "Greater Than 10 G Ohm"=10000000000.0] ("Configuration:Measurement Options:Input Resistance")
          n345 = property class="niDMM"(reference=w907, error in=w906, "Input Resistance"=w908) -> (reference out=w902:refnum<k15>, error out=w901:errorcluster)
          n346 = call-poly <instrlib>:"niDMM Config Measurement.vi"("Range"=-1.0, "Resolution in Digits"=w904, "error in (no error)"=w901, "Function"=niDMM_Function."DC Volts", "instrument handle"=w902) -> ("error out"=w899:errorcluster, "instrument handle out"=w900:refnum<k15>)  [unwired: 5 in]
        }
      }
    }
    frame Enabled {
    }
  }
  n347 = disable-structure shown="Enabled" {
    frame Disabled {
      n348 = case shown="15" {
        selector: _ -> [_ _]
        tunnel: _ -> [w910 w919]
        tunnel: _ -> [w909 w918]
        tunnel: [w910 w912] -> _
        tunnel: [w909 w911] -> _
        frame 0, Default {
        }
        frame 15 {
          w916 = T7 6.5 items=["3 1/2"=3.5, "4 1/2"=4.5, "5 1/2"=5.5, "6 1/2"=6.5, "7 1/2"=7.5] ("Resolution in Digits")
          w920 = 10000000000.0 items=["1 M Ohm"=1000000.0, "10 M Ohm"=10000000.0, "Greater Than 10 G Ohm"=10000000000.0] ("Configuration:Measurement Options:Input Resistance")
          n349 = property class="niDMM"(reference=w919, error in=w918, "Input Resistance"=w920) -> (reference out=w914:refnum<k15>, error out=w913:errorcluster)
          n350 = call-poly <instrlib>:"niDMM Config Measurement.vi"("Range"=-1.0, "Resolution in Digits"=w916, "error in (no error)"=w913, "Function"=niDMM_Function."DC Volts", "instrument handle"=w914) -> ("error out"=w911:errorcluster, "instrument handle out"=w912:refnum<k15>)  [unwired: 5 in]
        }
      }
    }
    frame Enabled {
    }
  }
  n351 = call <vilib>:"niSE Close Session.vi"("error in (no error)"=w8, "NISE Session (in)"=w7) -> ("error out"=→"error out":errorcluster)  [unwired: 5 in]
  n352 = call <instrlib>:"niDMM Close.vi"("error in (no error)"=w4, "instrument handle"=w5) -> ()  [unwired: 9 in, 1 out]
